vi "Engine Initialize.vi"(4 "Device Outputs FIFO":refnum<k33>, 6 "Device Inputs FIFO":refnum<k33>, 7 "Initialization Status Notifier":refnum<notifier>, 8 "error in (no error)":errorcluster, 11 "Device Reference":T8 format="%.0x") -> (0 "error out":errorcluster, 2 "Engine Run Time Data":T1, 3 "Device Reference Dup":T8 format="%.0x", 5 "Device Name":string)   [LabVIEW 2023, in "NI 272x Resistive Simulation Custom Device Engine.lvlib"]
uses:
  NI 272x Resistive Simulation Custom Device Engine.lvlib
  <vilib>/NI VeriStand/Custom Device API/Custom Device API.lvlib
  Globals/Names.vi
  NI 272x Resistive Simulation Custom Device Shared.lvlib
  Controls/Channel Mode.ctl
  <instrlib>/ni272xReferenceVIs/ni272xReferenceVIs.llb/ni272x Callendar-Van Dusen RTD Parameters.ctl
  Controls/Compiled HW Channel.ctl
  Controls/Compiled Connect Channel.ctl
  Controls/Compiled Engine Data.ctl
  Controls/Engine Run Time Data.ctl
  <vilib>/NI VeriStand/Custom Device Tools/Custom Device Utility Library/Custom Device Utility Library.lvlib
  <instrlib>/ni272xReferenceVIs/ni272xReferenceVIs.llb/ni272x Reference.ctl
  <vilib>/NI VeriStand/Custom Device API/Get Item Property (Variant).vi
  <vilib>/NI VeriStand/Custom Device API/Custom Device Item Ref.ctl
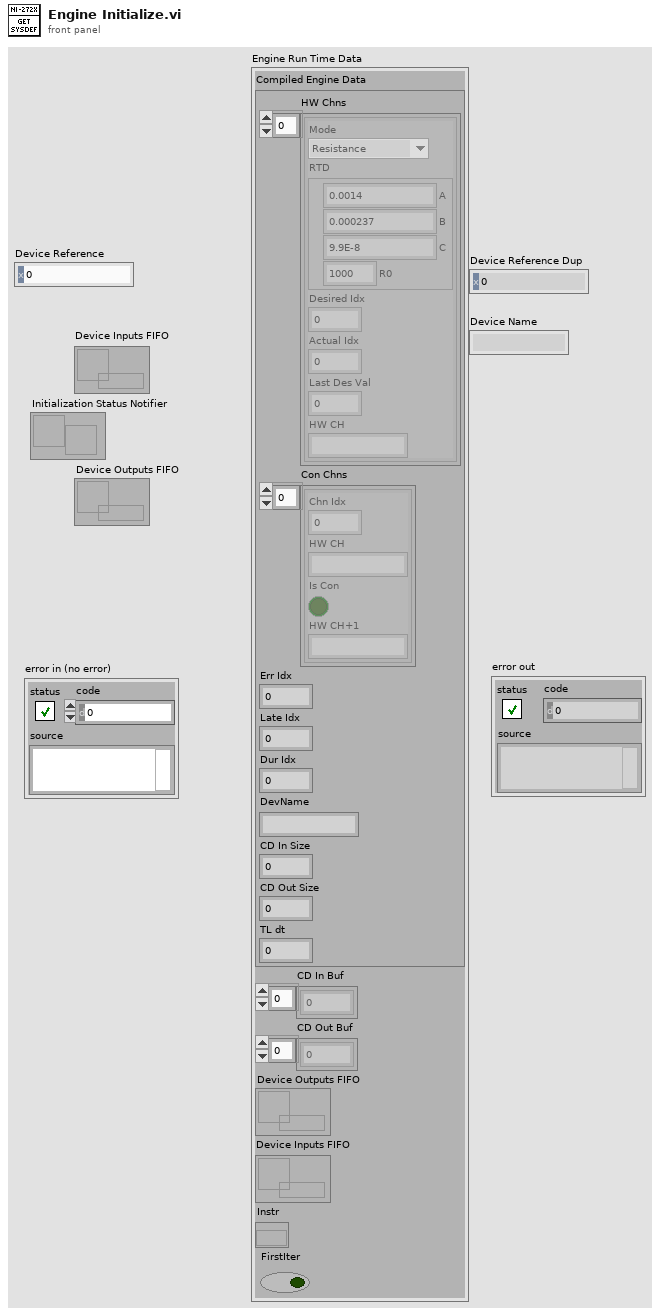
[diagram p1: front panel]
types:
  T1 = typedef "NI 272x Resistive Simulation Custom Device Engine.lvlib/Engine Run Time Data.ctl" = cluster{"Compiled Engine Data":T2, "CD In Buf":dbl[], "CD Out Buf":dbl[], "Device Outputs FIFO":refnum<k33>, "Device Inputs FIFO":refnum<k33>, "Instr":T7, "FirstIter":bool}
  T2 = typedef "NI 272x Resistive Simulation Custom Device Shared.lvlib/Compiled Engine Data.ctl" = cluster{"HW Chns":T3[], "Con Chns":T6[], "Err Idx":i32, "Late Idx":i32, "Dur Idx":i32, "DevName":string, "CD In Size":i32, "CD Out Size":i32, "TL dt":i64}
  T3 = typedef "NI 272x Resistive Simulation Custom Device Shared.lvlib/Compiled HW Channel.ctl" = cluster{"Mode":T4, "RTD":T5, "Desired Idx":i32, "Actual Idx":i32, "Last Des Val":dbl, "HW CH":string}
  T4 = typedef "NI 272x Resistive Simulation Custom Device Shared.lvlib/Channel Mode.ctl" = enum16{"Resistance", "RTD Temperature"}
  T5 = typedef "ni272x Callendar-Van Dusen RTD Parameters.ctl" = cluster{"A":dbl, "B":dbl, "C":dbl, "R0":dbl}
  T6 = typedef "NI 272x Resistive Simulation Custom Device Shared.lvlib/Compiled Connect Channel.ctl" = cluster{"Chn Idx":i32, "HW CH":string, "Is Con":bool, "HW CH+1":string}
  T7 = typedef "ni272x Reference.ctl" = refnum<k20>
  T8 = typedef "Custom Device API.lvlib/Custom Device Item Ref.ctl" = u64
  T9 = typedef "Custom Device API.lvlib/Custom Device Item Info.ctl" = cluster{"Name":string, "Is Channel":bool, "GUID":string, "Is Waveform":bool}
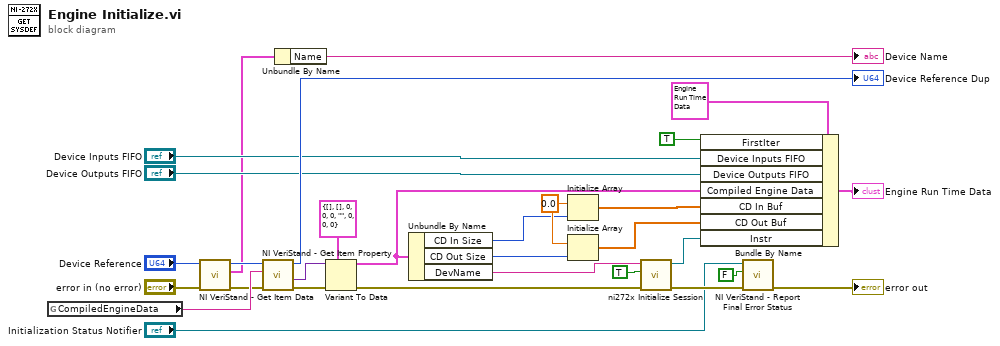
[diagram p0: block diagram]
diagram:
  w23 = 0.0 ("element")
  n1 = global read "Names.vi" "CompiledEngineData"() -> (w27:string)
  n2 = call <vilib>:"NI VeriStand - Get Item Data.vi"("error in (no error)"="error in (no error)", "Item Ref in"="Device Reference") -> ("error out"=w5:errorcluster, "Item Info"=w2:T9, "Item Ref out"=w3:T8)  [unwired: 6 in, 1 out]
  n3 = call-poly <vilib>:"NI VeriStand - Get Item Property.vi"("error in (no error)"=w5, "Property Name"=w27, "Item Ref in"=w3) -> ("error out"=w29:errorcluster, "Value"=w26:variant, "Item Ref out"=→"Device Reference Dup":T8)  [unwired: 5 in, 1 out]
  n4 = Unbundle By Name(w2) -> ("Name"=→"Device Name":string)
  n5 = Variant To Data(error in=w29, type=T2 {"HW Chns"=[], "Con Chns"=[], "Err Idx"=0, "Late Idx"=0, "Dur Idx"=0, "DevName"="", "CD In Size"=0, "CD Out Size"=0, "TL dt"=0} ("Compiled Engine Data"), Variant=w26) -> (data=w20:T2, error out=w13:errorcluster)
  n6 = Unbundle By Name(w20) -> ("CD In Size"=w22:i32, "CD Out Size"=w21:i32, "DevName"=w12:string)
  n7 = Initialize Array(w23, w22) -> (w19:dbl[])
  n8 = Initialize Array(w23, w21) -> (w18:dbl[])
  n9 = call <instrlib>:"ni272x Initialize Session.vi"("error in (no error)"=w13, "reset device (T)"=TRUE, "DAQmx Device Name"=w12) -> ("error out"=w11:errorcluster, "instrument handle out"=w7:T7)  [unwired: 7 out]
  n10 = Bundle By Name(cluster=T1 {"Compiled Engine Data"={"HW Chns"=[], "Con Chns"=[], "Err Idx"=0, "Late Idx"=0, "Dur Idx"=0, "DevName"="", "CD In Size"=0, "CD Out Size"=0, "TL dt"=0}, "CD In Buf"=[], "CD Out Buf"=[], "Device Outputs FIFO"=refnum, "Device Inputs FIFO"=refnum, "Instr"=refnum, "FirstIter"=FALSE} ("Engine Run Time Data"), "FirstIter"=TRUE, "Device Inputs FIFO"="Device Inputs FIFO", "Device Outputs FIFO"="Device Outputs FIFO", "Compiled Engine Data"=w20, "CD In Buf"=w19, "CD Out Buf"=w18, "Instr"=w7) -> (→"Engine Run Time Data":T1)
  n11 = call <vilib>:"NI VeriStand - Report Final Error Status.vi"("error in (no error)"=w11, "Filter FIFO & Shutdown Errors (T)"=FALSE ("Filter FIFO Errors (T)"), "Status Notifier"="Initialization Status Notifier") -> ("error out"=→"error out":errorcluster)  [unwired: 8 out]
